vi "Set Row Col of Direction.vi"(7 "Direction":T1, 10 "Column":i32, 11 "Row":i32) -> (2 "Col Direction":i32, 3 "Row Direction":i32)   [LabVIEW 2016, in "AntFarm_MB.lvclass"]
uses:
  AntFarm_MB.lvclass
  Type Defs/Direction Enum.ctl
  SubVIs/Read-Only Globals.vi
  SubVIs/Globals (private).vi
  Square/Square.lvclass
  Type Defs/SB Type Defs.lvlib
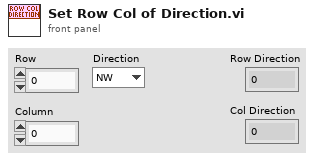
[diagram p1: front panel]
types:
  T1 = typedef "SB Type Defs.lvlib/Direction Enum.ctl" = enum16{"NW", "N", "NE", "E", "SE", "S", "SW", "W"}
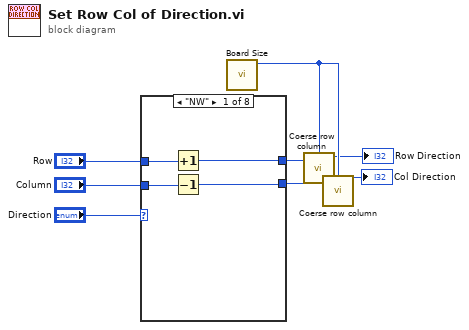
[diagram p0: block diagram]
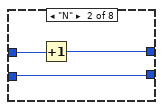
[diagram p2: hidden frame]
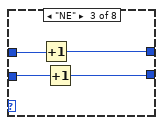
[diagram p3: hidden frame]
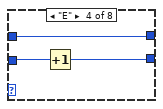
[diagram p4: hidden frame]
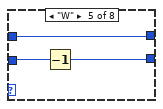
[diagram p5: hidden frame]
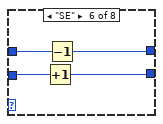
[diagram p6: hidden frame]
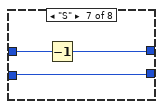
[diagram p7: hidden frame]
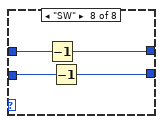
[diagram p8: hidden frame]
diagram:
  n1 = case shown="\"NW\"" "Direction" {
    tunnel: "Column" -> [w11 w13 w17 w22 w25 w29 w30 w34]
    tunnel: "Row" -> [w12 w15 w19 w20 w23 w27 w32 w36]
    tunnel: [w10 w14 w18 w20 w23 w26 w31 w35] -> w4
    tunnel: [w9 w13 w16 w21 w24 w28 w30 w33] -> w6
    frame "NW" {
      n2 = Increment(x=w12) -> (x+1=w10:i32)
      n3 = Decrement(x=w11) -> (x-1=w9:i32)
    }
    frame "N" {
      n4 = Increment(x=w15) -> (x+1=w14:i32)
    }
    frame "NE" {
      n5 = Increment(x=w19) -> (x+1=w18:i32)
      n6 = Increment(x=w17) -> (x+1=w16:i32)
    }
    frame "E" {
      n7 = Increment(x=w22) -> (x+1=w21:i32)
    }
    frame "W" {
      n8 = Decrement(x=w25) -> (x-1=w24:i32)
    }
    frame "SE" {
      n9 = Increment(x=w29) -> (x+1=w28:i32)
      n10 = Decrement(x=w27) -> (x-1=w26:i32)
    }
    frame "S" {
      n11 = Decrement(x=w32) -> (x-1=w31:i32)
    }
    frame "SW" {
      n12 = Decrement(x=w36) -> (x-1=w35:i32)
      n13 = Decrement(x=w34) -> (x-1=w33:i32)
    }
  }
  n14 = call "Board Size.vi"() -> ("Board Size"=w8:i32)  [unwired: 11 in]
  n15 = call "Coerse row column.vi"("Row Col"=w4, "Board Size"=w8) -> ("Coerced Out"=→"Row Direction":i32)  [unwired: 3 in]
  n16 = call "Coerse row column.vi"("Row Col"=w6, "Board Size"=w8) -> ("Coerced Out"=→"Col Direction":i32)  [unwired: 3 in]
